vi "Counter - Read Encoder Velocity (Continuous Clock).vi"() -> ()   [LabVIEW 2015]
doc: "This example demonstrates how to use a counter input along with an external clock to continually sample the angular velocity measured from an encoder.\n\nFor instructions on how to connect your signals to the DAQ device, refer to your device documentation."
uses:
  <vilib>/Utility/error.llb/DialogType.ctl
  <vilib>/DAQmx/read.llb/DAQmx Read (Counter 2D DBL NChan NSamp).vi
  <vilib>/DAQmx/create/channels.llb/DAQmx Create Channel (CI-Frequency).vi
  <vilib>/DAQmx/create/channels.llb/DAQmx Create Channel (CI-Position-Angular Encoder).vi
  <vilib>/DAQmx/configure/timing.llb/DAQmx Timing (Sample Clock).vi
  <vilib>/DAQmx/miscellaneous.llb/DAQmx Fill In Error Info.vi
  <resource>/objmgr/daqmx.rc
panel:
  in  "Counter 0":tag="cDAQ1Mod4/ctr0"
  in  "Min Frequency":dbl=2.0 format="%0.6f"
  in  "Max Frequency":dbl=100.0 format="%0.6f"
  in  "Frequency Input Terminal":tag="PFI0"
  in  "Z Index Terminal":tag="PFI2"
  in  "Z Index Enable":bool
  in  "Pulses Per Revolution":u32=24
  in  "B Input Terminal":tag="PFI1"
  in  "A Input Terminal":tag="PFI0"
  in  "Counter 1":tag="cDAQ1Mod4/ctr1"
  in  "Trigger Type":enum32{"No Trigger", "Digital Arm Start"}(tab)
  in  "Edge":i32(ring)=10280 items=["Rising"=10280, "Falling"=10171]
  in  "Digital Trigger Source":tag
  out "Acquired Data":dbl[](array[numeric])
  in  "Stop":bool
  in  "Samples per Loop":i32=100
  in  "Sample Rate":dbl=1000.0
  in  "Sample Clock Source":tag="OnboardClock"
  # "Acquired Data\nPulses/Second"
  # "Channel Settings"
  # "Timing Settings"
  # "Trigger Settings"
  # "To configure and use a trigger or the count reset you must have the necessary tab selected above.  Not all hardware supports the above options--refer to your device documentation for more info."
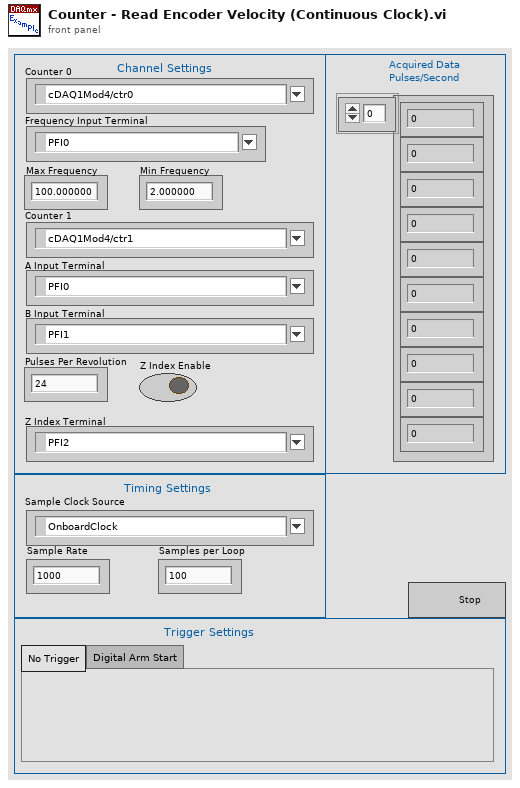
[diagram p1: front panel]
types:
  T1 = typedef "DialogType.ctl" = u16
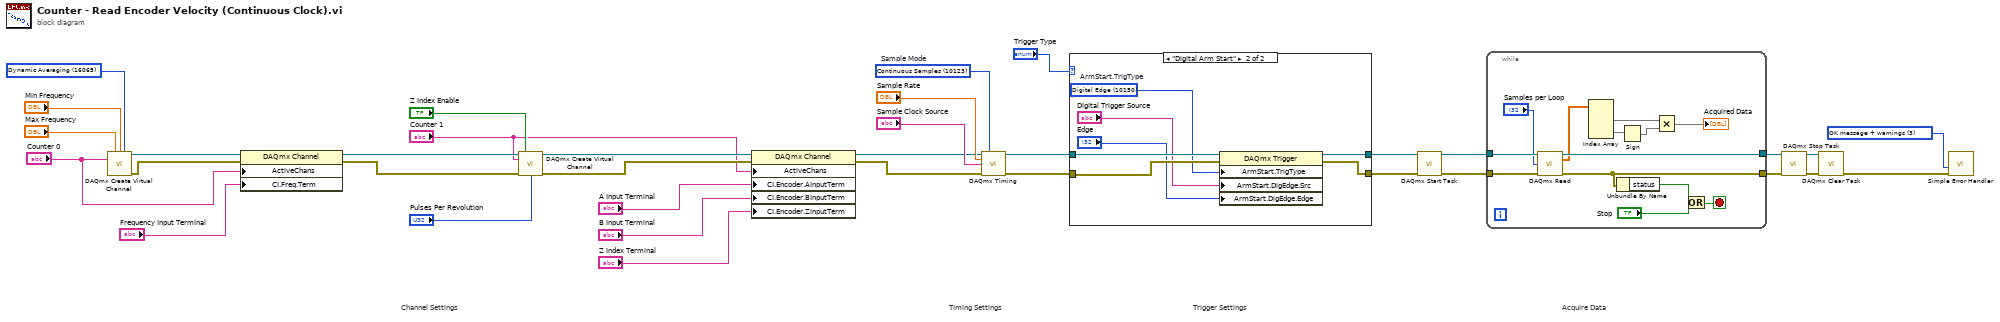
[diagram p0: block diagram]
diagram:
  w1 = 16065 items=["Low Frequency with 1 Counter"=10105, "High Frequency with 2 Counters"=10157, "Large Range with 2 Counters"=10205, "Dynamic Averaging"=16065] ("measurement method")
  w12 = T1 3 items=["no dialog", "OK message", "continue or stop message", "OK message + warnings", "continue/stop + warnings"] ("type of dialog (OK msg:1)")
  w35 = 10123 items=["Finite Samples"=10178, "Continuous Samples"=10123, "Hardware Timed Single Point"=12522]  # Sample Mode
  # "Acquire Data"
  # "Trigger Settings"
  # "Timing Settings"
  # "Channel Settings"
  n1 = call-poly <vilib>:"DAQmx Create Virtual Channel.vi"("maximum value"="Max Frequency", "minimum value"="Min Frequency", "measurement method"=w1, "counter"="Counter 0") -> ("task out"=w11:refnum<k21>, "error out"=w10:errorcluster)  [unwired: 10 in]
  n2 = property class="DAQmx Channel"(reference=w11, error in=w10, "ActiveChans"="Counter 0", "CI.Freq.Term"="Frequency Input Terminal") -> (reference out=w7:refnum<k21>, error out=w6:errorcluster)
  n3 = call-poly <vilib>:"DAQmx Create Virtual Channel.vi"("task in"=w7, "z index enable"="Z Index Enable", "counter"="Counter 1", "error in"=w6, "pulses per revolution"="Pulses Per Revolution") -> ("task out"=w24:refnum<k21>, "error out"=w23:errorcluster)  [unwired: 9 in]
  n4 = property class="DAQmx Channel"(reference=w24, error in=w23, "ActiveChans"="Counter 1", "CI.Encoder.AInputTerm"="A Input Terminal", "CI.Encoder.BInputTerm"="B Input Terminal", "CI.Encoder.ZInputTerm"="Z Index Terminal") -> (reference out=w19:refnum<k21>, error out=w18:errorcluster)
  n5 = call-poly <vilib>:"DAQmx Timing.vi"("task/channels in"=w19, "sample mode"=w35, "rate"="Sample Rate", "source"="Sample Clock Source", "error in"=w18) -> ("task out"=w26:refnum<k21>, "error out"=w25:errorcluster)  [unwired: 9 in]
  n6 = case shown="\"Digital Arm Start\"" "Trigger Type" {
    tunnel: w26 -> [w37 w44]
    tunnel: w25 -> [w36 w41]
    tunnel: [w37 w43] -> w27
    tunnel: [w36 w42] -> w28
    frame "No Trigger", Default {
    }
    frame "Digital Arm Start" {
      w38 = 10150 items=["Digital Edge"=10150, "None"=10230]  # ArmStart.TrigType
      n7 = property class="DAQmx Trigger"(reference=w44, error in=w41, "ArmStart.TrigType"=w38, "ArmStart.DigEdge.Src"="Digital Trigger Source", "ArmStart.DigEdge.Edge"="Edge") -> (reference out=w43:refnum<k21>, error out=w42:errorcluster)
    }
  }
  n8 = call <vilib>:"DAQmx Start Task.vi"("task/channels in"=w27, "error in"=w28) -> ("task out"=w34:refnum<k21>, "error out"=w33:errorcluster)  [unwired: 12 in]
  n9 = while {
    tunnel: w34 -> [w57]
    tunnel: w33 -> [w56]
    tunnel: [w53] -> w15
    tunnel: [w54] -> w16
    stop <- w55 stop-if-true
    n10 = call-poly <vilib>:"DAQmx Read.vi"("task/channels in"=w57, "number of samples per channel"="Samples per Loop", "error in"=w56) -> ("task out"=w54:refnum<k21>, "data"=w49:dbl[][], "error out"=w53:errorcluster)  [unwired: 10 in]
    n11 = Index Array(array=w49) -> (element #1=w47:dbl[], element #2=w48:dbl[])  [unwired: 4 in]
    n12 = Unbundle By Name(w53) -> ("status"=w52:bool)
    n13 = Sign(1:w48) -> (0:w46:dbl[])
    n14 = Multiply(x=w47, y=w46) -> (x*y=→"Acquired Data":dbl[])
    n15 = Or(x=w52, y="Stop") -> (x .or. y?=w55:bool)
  }
  n16 = call <vilib>:"DAQmx Stop Task.vi"("task/channels in"=w16, "error in"=w15) -> ("task out"=w13:refnum<k21>, "error out"=w14:errorcluster)  [unwired: 12 in]
  n17 = call <vilib>:"DAQmx Clear Task.vi"("task in"=w13, "error in"=w14) -> ("error out"=w32:errorcluster)  [unwired: 13 in]
  n18 = call <vilib>:"Simple Error Handler.vi"("type of dialog (OK msg:1)"=w12, "error in (no error)"=w32) -> ()  [unwired: 3 in, 5 out]
